vi "2D Inverse Real FFT.vi"(10 "shift?":bool, 11 "FFT {X}":cdb[][](array[numeric])) -> (0 "error":i32, 3 "X":dbl[][](array[numeric]))   [LabVIEW 2010, in "NI_AALPro.lvlib"]
doc: "Computes the inverse discrete Fourier transform (IDFT) of the input sequence <B>FFT {X}</B>. You must manually select the polymorphic instance you want to use."
uses:
  NI_AALPro.lvlib
  lvanlys.dll
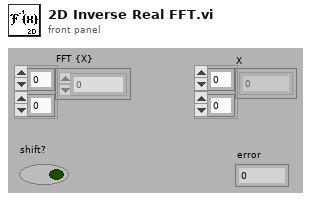
[diagram p1: front panel]
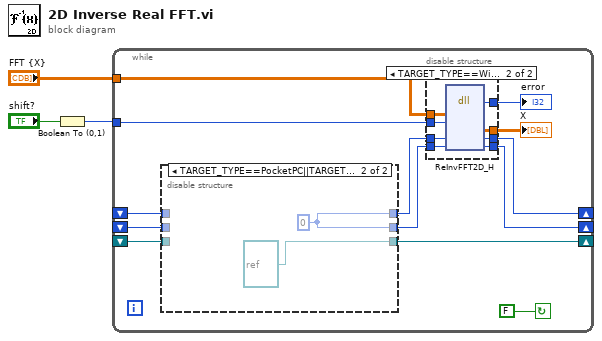
[diagram p0: block diagram]
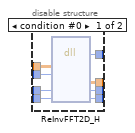
[diagram p2: hidden frame]
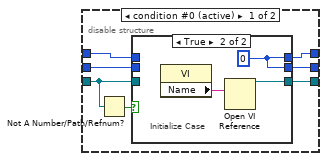
[diagram p3: hidden frame]
diagram:
  n1 = Boolean To (0,1)(Boolean="shift?") -> (0, 1=w1:i16)
  n2 = while {
    shift-left: _ -> [w14]
    shift-right: [w8] -> _
    tunnel: "FFT {X}" -> [w15]
    shift-right: [w13] -> _
    shift-left: _ -> [w12]
    shift-right: [w7] -> _
    shift-left: _ -> [w11]
    tunnel: w1 -> [w4]
    stop <- FALSE continue-if-true
    n3 = disable-structure shown="TARGET_TYPE==PocketPC||TARGET_TYPE==PalmOS||TARGET_TYPE==FPGA||TARGET_TYPE==Embedded" {
      disable-tunnel: w12 -> [w37 _]
      disable-tunnel: [w38 refnum<vi> refnum ("VI Refnum")] -> w13
      disable-tunnel: w14 -> [w36 _]
      disable-tunnel: [w35 w47] -> w9
      disable-tunnel: [w34 w47] -> w6
      disable-tunnel: w11 -> [w33 _]
      frame condition #0 (active) {
        n4 = Not A Number/Path/Refnum?(number/path/refnum=w37) -> (NaN/Path/Refnum?=w39:bool)
        n5 = case shown="True" w39 {
          tunnel: [w42 w44] -> w38
          tunnel: w37 -> [w42 _]
          tunnel: w36 -> [w41 _]
          tunnel: [w41 w45] -> w35
          tunnel: [w40 w45] -> w34
          tunnel: w33 -> [w40 _]
          frame False {
          }
          frame True {
            w45 = 0 ("error")
            # "Initialize Case"
            n6 = property class="VI"() -> ("Name"=w43:string)  [unwired: 2 in, 2 out]
            n7 = Open VI Reference(vi path=w43) -> (vi reference=w44:refnum<vi>)  [unwired: 5 in, 1 out]
          }
        }
      }
      frame condition #1 {
        w47 = 0 ("t")
      }
    }
    n8 = disable-structure shown="TARGET_TYPE==Windows||TARGET_TYPE==Mac||TARGET_TYPE==Unix" {
      disable-tunnel: w15 -> [w24 w32]
      disable-tunnel: [w23 w31] -> w10
      disable-tunnel: w9 -> [w22 w30]
      disable-tunnel: [w21 w29] -> w8
      disable-tunnel: [w20 w28] -> w7
      disable-tunnel: w6 -> [w19 w27]
      disable-tunnel: [w18 w26] -> w5
      disable-tunnel: w4 -> [w17 w25]
      frame condition #0 {
        n9 = dll-call lib="C:/Program Files/National Instruments/LabVIEW 2010/resource/lvanlys.dll" fn="ReInvFFT2D_H"("xH"=w24, "shifted"=w17, "tblRow"=w22, "tblCol"=w19) -> ("return type"=w23:i32, "yH"=w18:dbl[][], "tblRow"=w21:i32, "tblCol"=w20:i32)  [unwired: 6 in, 2 out]
      }
      frame condition #1 (active) {
        n10 = dll-call lib="C:/Program Files/National Instruments/LabVIEW 2010/resource/lvanlys.dll" fn="ReInvFFT2D_H"("xH"=w32, "shifted"=w25, "tblRow"=w30, "tblCol"=w27) -> ("return type"=w31:i32, "yH"=w26:dbl[][], "tblRow"=w29:i64, "tblCol"=w28:i64)  [unwired: 6 in, 2 out]
      }
    }
    "X" <- w5
    "error" <- w10
  }
